vi "Get Path to Latest Installer.vi"(8 "error in (no error)":errorcluster, 11 "SelfUpdate in":refnum<class "SelfUpdate.lvclass">) -> (0 "error out":errorcluster, 2 "Path to download":string, 3 "SelfUpdate out":refnum<class "SelfUpdate.lvclass">)   [LabVIEW 2013, in "SelfUpdate.lvclass"]
uses:
  SelfUpdate.lvclass
  <vilib>/addons/_JKI.lib/REST Client/classes/REST Client/REST Client.lvclass
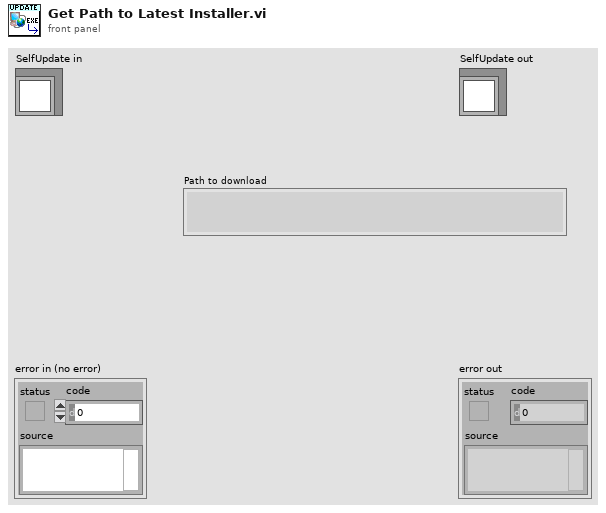
[diagram p1: front panel]
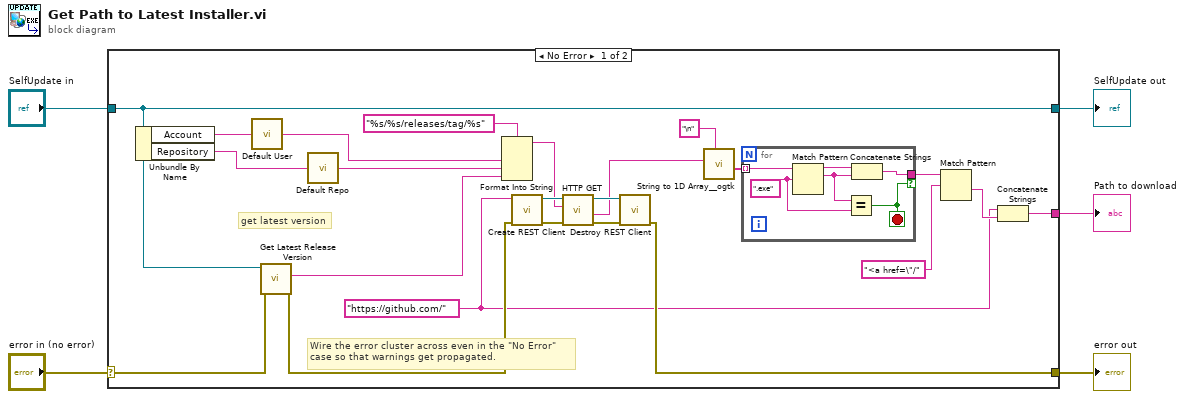
[diagram p0: block diagram]
diagram:
  n1 = case shown="No Error" "error in (no error)" {
    selector: "error in (no error)" -> [w21 w36]
    tunnel: [w24 w36] -> w4
    tunnel: [w23 w35] -> w2
    tunnel: "SelfUpdate in" -> [w23 w35]
    tunnel: [w9 _] -> w1
    frame No Error {
      w10 = "https://github.com/" ("format string")
      # "get latest version"
      # "Wire the error cluster across even in the \"No Error\"\ncase so that warnings get propagated."
      n2 = Unbundle By Name(w23) -> ("Account"=w28:string, "Repository"=w8:string)
      n3 = call "Default User.vi"("Account in"=w28) -> ("Account out"=w6:string)
      n4 = call "Get Latest Release Version.vi"("error in (no error)"=w21, "SelfUpdate in"=w23) -> ("error out"=w20:errorcluster, "latest tag"=w19:string)  [unwired: 7 in, 1 out]
      n5 = call "Default Repo.vi"("Repo in"=w8) -> ("Repo out"=w7:string)
      n6 = Format Into String(format string="%s/%s/releases/tag/%s", w6, w7, w19) -> (resulting string=w16:string)  [unwired: 2 in, 1 out]
      n7 = call <vilib>:"Create REST Client.vi"("error in (no error)"=w20, "Base URL"=w10) -> ("error out"=w25:errorcluster, "REST Client out"=w26:refnum<class "REST Client.lvclass">)  [unwired: 8 in]
      n8 = call-dynamic "HTTP GET.vi"("error in (no error)"=w25, "Path"=w16, "REST Client in"=w26) -> ("error out"=w18:errorcluster, "Response body"=w17:string, "REST Client out"=w27:refnum<class "REST Client.lvclass">)  [unwired: 3 in, 3 out]
      n9 = call-dynamic "Destroy REST Client.vi"("error in (no error)"=w18, "REST Client in"=w27) -> ("error out"=w24:errorcluster)  [unwired: 9 in]
      n10 = call "String to 1D Array__ogtk.vi"("delimiter (Tab)"="\n", "string"=w17) -> ("Array of Strings"=w15:string[])  [unwired: 9 in]
      n11 = for {
        tunnel: w15 -> [w32] mode=indexing
        tunnel: [w29] -> w13 if=w33
        stop <- w33 stop-if-true
        w34 = ".exe" ("regular expression")
        n12 = Match Pattern(string=w32, regular expression=w34) -> (before substring=w31:string, match substring=w30:string)  [unwired: 1 in, 2 out]
        n13 = Equal?(x=w30, y=w34) -> (x = y?=w33:bool)
        n14 = Concatenate Strings(w31, w30) -> (w29:string)
      }
      n15 = Match Pattern(string=w13, regular expression="<a href=\"/") -> (after substring=w11:string)  [unwired: 1 in, 3 out]
      n16 = Concatenate Strings(w10, w11) -> (w9:string)
    }
    frame Error {
    }
  }
  "error out" <- w4
  "SelfUpdate out" <- w2
  "Path to download" <- w1
